vi "map modbus addresses test.vi"() -> ()   [LabVIEW 2013, in "Modbus Slave tests.lvlib"]
uses:
  Modbus Slave tests.lvlib
  configuration/Modbus Slave configuration.lvclass
  configuration/modbus mapping behavior.ctl
  <vilib>/NI/Tag Bus Module Framework/channel/channel classification.ctl
  <vilib>/NI/Tag Bus/tag/Data Type.ctl
  module channel/data bank type.ctl
  module channel/Modbus Module Channel.lvclass
  <vilib>/NI/Tag Bus/tag/tag descriptor.lvclass/tag descriptor.ctl
  <vilib>/NI/Tag Bus Module Framework/channel/TBM channel.lvclass/TBM channel.ctl
  module channel/Modbus Module Channel.lvclass/Modbus Module Channel.ctl
  configuration/Modbus Slave configuration.lvclass/Modbus Slave configuration.ctl
  <vilib>/NI/Tag Bus/tag/write tag name.vi
  <vilib>/NI/Tag Bus Module Framework/channel/Write channel classification.vi
  <vilib>/NI/Tag Bus/tag/write data type.vi
  module channel/Write modbus type.vi
  module channel/Write starting address.vi
  module channel/Write subindex (bool).vi
  <vilib>/NI/Tag Bus/tag/read tag name.vi
  <vilib>/NI/Tag Bus Module Framework/channel/Read channel classification.vi
  <vilib>/NI/Tag Bus/tag/read data type.vi
  module channel/Read modbus type.vi
  module channel/Read starting address.vi
  module channel/Read subindex (bool).vi
  <vilib>/NI/Tag Bus Module Framework/channel/TBM channel.lvclass
  <vilib>/NI/Tag Bus/tag/tag descriptor.lvclass
panel:
  in  "CSV Test File Path":path
  out "error out":errorcluster
  out "OK":bool
  in  "error in":errorcluster
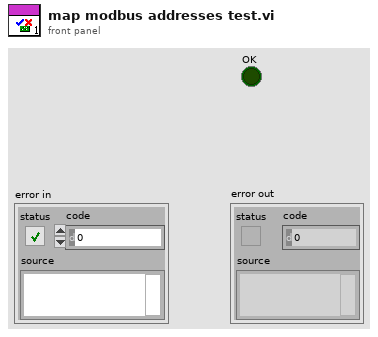
[diagram p1: front panel]
types:
  T1 = typedef "TBM channel.lvclass/channel classification.ctl" = enum16{"input data", "output data", "processing parameter", "processing result"}
  T2 = typedef "tag bus.lvlib/tag descriptor.lvclass/Data Type.ctl" = enum16{"Double", "Single", "I64", "I32", "I16", "I8", "U64", "U32", "U16", "U8", "Boolean", "String", "Array of Double", "Array of Single", "Array of I64", "Array of I32", "Array of I16", "Array of I8", "Array of U64", "Array of U32", "Array of U16", "Array of U8", "Array of Boolean", "Array of String"}
  T3 = typedef "Modbus Module Channel.lvclass/data bank type.ctl" = enum16{"coils", "discrete inputs", "input registers", "holding registers"}
  T4 = cluster{"name":string, "channel classification":T1, "data type":T2, "modbus type":T3, "starting address":u16, "subindex (bool)":i32}[]
  T5 = typedef "Modbus Slave configuration.lvclass/modbus mapping behavior.ctl" = enum16{"custom", "optimized"}
  T6 = cluster{"name":string, "channel classification":T1, "data type":T2, "modbus type":T3, "starting address":u16, "subindex (bool)":i32}
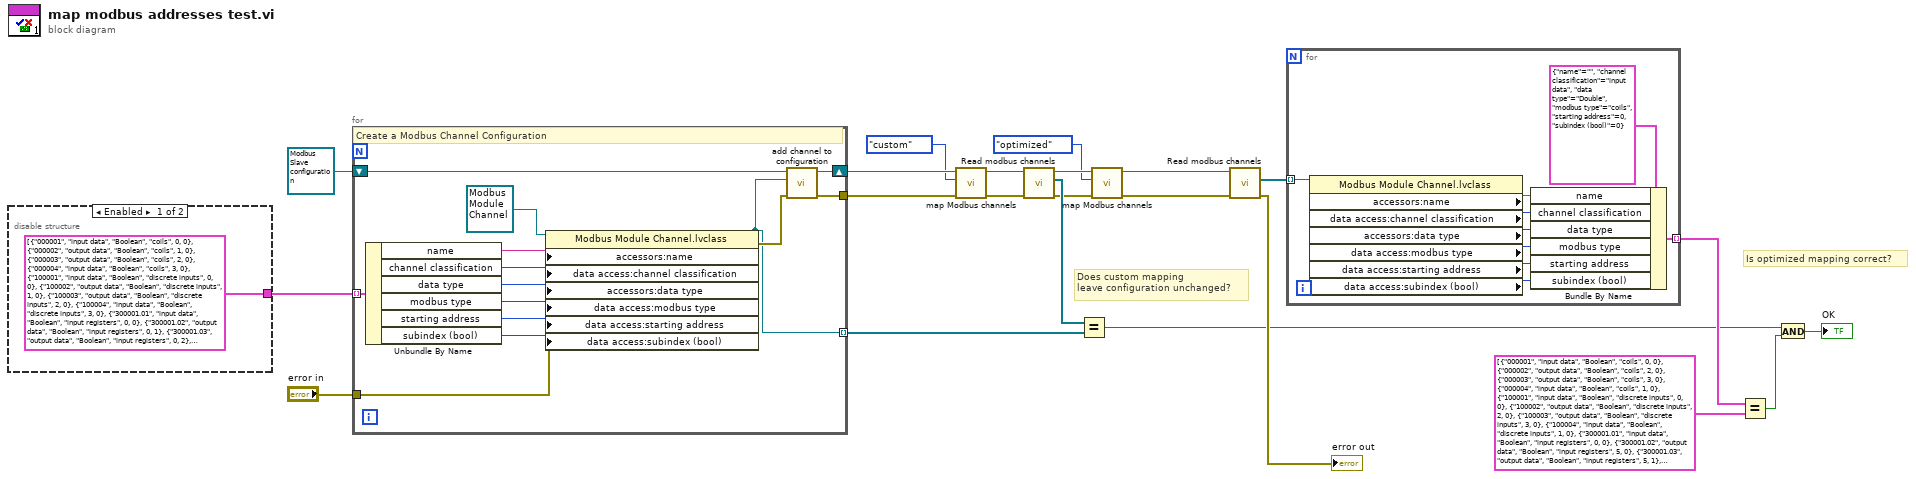
[diagram p0: block diagram]
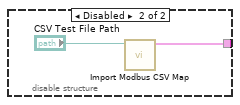
[diagram p2: hidden frame]
diagram:
  # "Is optimized mapping correct?"
  # "Does custom mapping\nleave configuration unchanged?"
  n1 = disable-structure shown="Enabled" {
    disable-tunnel: [T4 [{"name"="000001", "channel classification"=enum."input data", "data type"=enum."Boolean", "modbus type"=enum."coils", "starting address"=0, "subindex (bool)"=0}, {"name"="000002", "channel classification"=enum."output data", "data type"=enum."Boolean", "modbus type"=enum."coils", "starting address"=1, "subindex (bool)"=0}, {"name"="000003", "channel classification"=enum."output data", "data type"=enum."Boolean", "modbus type"=enum."coils", "starting address"=2, "subindex (bool)"=0}, {"name"="000004", "channel classification"=enum."input data", "data type"=enum."Boolean", "modbus type"=enum."coils", "starting address"=3, "subindex (bool)"=0}, {"name"="100001", "channel classification"=enum."input data", "data type"=enum."Boolean", "modbus type"=enum."discrete inputs", "starting address"=0, "subindex (bool)"=0}, {"name"="100002", "channel classification"=enum."output data", "data type"=enum."Boolean", "modbus type"=enum."discrete inputs", "starting address"=1, "subindex (bool)"=0}, {"name"="100003", "channel classification"=enum."output data", "data type"=enum."Boolean", "modbus type"=enum."discrete inputs", "starting address"=2, "subindex (bool)"=0}, {"name"="100004", "channel classification"=enum."input data", "data type"=enum."Boolean", "modbus type"=enum."discrete inputs", "starting address"=3, "subindex (bool)"=0}, {"name"="300001.01", "channel classification"=enum."input data", "data type"=enum."Boolean", "modbus type"=enum."input registers", "starting address"=0, "subindex (bool)"=0}, {"name"="300001.02", "channel classification"=enum."output data", "data type"=enum."Boolean", "modbus type"=enum."input registers", "starting address"=0, "subindex (bool)"=1}, {"name"="300001.03", "channel classification"=enum."output data", "data type"=enum."Boolean", "modbus type"=enum."input registers", "starting address"=0, "subindex (bool)"=2}, {"name"="300001.04", "channel classification"=enum."input data", "data type"=enum."Boolean", "modbus type"=enum."input registers", "starting address"=0, "subindex (bool)"=3}, {"name"="300001", "channel classification"=enum."input data", "data type"=enum."Single", "modbus type"=enum."input registers", "starting address"=0, "subindex (bool)"=0}, {"name"="300002", "channel classification"=enum."output data", "data type"=enum."Single", "modbus type"=enum."input registers", "starting address"=1, "subindex (bool)"=0}, {"name"="300003", "channel classification"=enum."output data", "data type"=enum."Single", "modbus type"=enum."input registers", "starting address"=2, "subindex (bool)"=0}, {"name"="300004", "channel classification"=enum."input data", "data type"=enum."Single", "modbus type"=enum."input registers", "starting address"=3, "subindex (bool)"=0}, {"name"="400001.01", "channel classification"=enum."input data", "data type"=enum."Boolean", "modbus type"=enum."holding registers", "starting address"=0, "subindex (bool)"=0}, {"name"="400001.02", "channel classification"=enum."output data", "data type"=enum."Boolean", "modbus type"=enum."holding registers", "starting address"=0, "subindex (bool)"=1}, {"name"="400001.03", "channel classification"=enum."output data", "data type"=enum."Boolean", "modbus type"=enum."holding registers", "starting address"=0, "subindex (bool)"=2}, {"name"="400001.04", "channel classification"=enum."input data", "data type"=enum."Boolean", "modbus type"=enum."holding registers", "starting address"=0, "subindex (bool)"=3}, {"name"="400001", "channel classification"=enum."input data", "data type"=enum."Double", "modbus type"=enum."holding registers", "starting address"=0, "subindex (bool)"=0}, {"name"="400002", "channel classification"=enum."output data", "data type"=enum."Double", "modbus type"=enum."holding registers", "starting address"=1, "subindex (bool)"=0}, {"name"="400003", "channel classification"=enum."output data", "data type"=enum."Double", "modbus type"=enum."holding registers", "starting address"=2, "subindex (bool)"=0}, {"name"="400004", "channel classification"=enum."input data", "data type"=enum."Double", "modbus type"=enum."holding registers", "starting address"=3, "subindex (bool)"=0}] ("Modbus address map 2") w25] -> w2
    frame Enabled {
    }
    frame Disabled {
      n2 = call "Import Modbus CSV Map.vi"("CSV Test File Path"="CSV Test File Path") -> ("Modbus address map"=w25:T4)  [unwired: 10 in]
    }
  }
  n3 = for {
    shift-right: [w29] -> w20
    shift-left: refnum<class "Modbus Slave configuration.lvclass"> refnum ("Modbus Slave configuration") -> [w31]
    tunnel: w2 -> [w38] mode=indexing
    tunnel: "error in" -> [w28]
    tunnel: [w27] -> w19
    tunnel: [w26] -> w14 mode=indexing
    # "Create a Modbus Channel Configuration"
    n4 = Unbundle By Name(w38) -> ("name"=w32:string, "channel classification"=w33:T1, "data type"=w34:T2, "modbus type"=w35:T3, "starting address"=w36:u16, "subindex (bool)"=w37:i32)
    n5 = property class="Modbus Module Channel.lvclass"(reference=refnum<class "Modbus Module Channel.lvclass"> refnum ("Modbus Module Channel.lvclass"), error in=w28, "accessors:name"=w32, "data access:channel classification"=w33, "accessors:data type"=w34, "data access:modbus type"=w35, "data access:starting address"=w36, "data access:subindex (bool)"=w37) -> (reference out=w26:refnum<class "Modbus Module Channel.lvclass">, error out=w30:errorcluster)
    n6 = call "add channel to configuration.vi"("error in"=w30, "Modbus Module Channel.lvclass"=w26, "Modbus Slave configuration in"=w31) -> ("error out"=w27:errorcluster, "Modbus Slave configuration out"=w29:refnum<class "Modbus Slave configuration.lvclass">)  [unwired: 7 in]
  }
  n7 = call "map Modbus channels.vi"("error in"=w19, "mapping"=modbus_mapping_behavior."custom", "Modbus Slave configuration in"=w20) -> ("error out"=w16:errorcluster, "Modbus Slave configuration out"=w17:refnum<class "Modbus Slave configuration.lvclass">)  [unwired: 7 in]
  n8 = call "Read modbus channels.vi"("error in"=w16, "Modbus Slave configuration in"=w17) -> ("error out"=w12:errorcluster, "modbus channels"=w15:refnum<class "Modbus Module Channel.lvclass">[], "Modbus Slave configuration out"=w13:refnum<class "Modbus Slave configuration.lvclass">)  [unwired: 7 in]
  n9 = Equal?(x=w15, y=w14) -> (x = y?=w5:bool)
  n10 = call "map Modbus channels.vi"("error in"=w12, "mapping"=modbus_mapping_behavior."optimized", "Modbus Slave configuration in"=w13) -> ("error out"=w9:errorcluster, "Modbus Slave configuration out"=w10:refnum<class "Modbus Slave configuration.lvclass">)  [unwired: 7 in]
  n11 = call "Read modbus channels.vi"("error in"=w9, "Modbus Slave configuration in"=w10) -> ("error out"=→"error out":errorcluster, "modbus channels"=w8:refnum<class "Modbus Module Channel.lvclass">[])  [unwired: 7 in, 1 out]
  n12 = for {
    tunnel: w8 -> [w48] mode=indexing
    tunnel: [w40] -> w6 mode=indexing
    n13 = property class="Modbus Module Channel.lvclass"(reference=w48) -> ("accessors:name"=w46:string, "data access:channel classification"=w45:T1, "accessors:data type"=w44:T2, "data access:modbus type"=w43:T3, "data access:starting address"=w42:u16, "data access:subindex (bool)"=w41:i32)  [unwired: 1 in, 2 out]
    n14 = Bundle By Name(cluster=T6 {"name"="", "channel classification"=enum."input data", "data type"=enum."Double", "modbus type"=enum."coils", "starting address"=0, "subindex (bool)"=0}, "name"=w46, "channel classification"=w45, "data type"=w44, "modbus type"=w43, "starting address"=w42, "subindex (bool)"=w41) -> (w40:T6)
  }
  n15 = Equal?(x=w6, y=T4 [{"name"="000001", "channel classification"=enum."input data", "data type"=enum."Boolean", "modbus type"=enum."coils", "starting address"=0, "subindex (bool)"=0}, {"name"="000002", "channel classification"=enum."output data", "data type"=enum."Boolean", "modbus type"=enum."coils", "starting address"=2, "subindex (bool)"=0}, {"name"="000003", "channel classification"=enum."output data", "data type"=enum."Boolean", "modbus type"=enum."coils", "starting address"=3, "subindex (bool)"=0}, {"name"="000004", "channel classification"=enum."input data", "data type"=enum."Boolean", "modbus type"=enum."coils", "starting address"=1, "subindex (bool)"=0}, {"name"="100001", "channel classification"=enum."input data", "data type"=enum."Boolean", "modbus type"=enum."discrete inputs", "starting address"=0, "subindex (bool)"=0}, {"name"="100002", "channel classification"=enum."output data", "data type"=enum."Boolean", "modbus type"=enum."discrete inputs", "starting address"=2, "subindex (bool)"=0}, {"name"="100003", "channel classification"=enum."output data", "data type"=enum."Boolean", "modbus type"=enum."discrete inputs", "starting address"=3, "subindex (bool)"=0}, {"name"="100004", "channel classification"=enum."input data", "data type"=enum."Boolean", "modbus type"=enum."discrete inputs", "starting address"=1, "subindex (bool)"=0}, {"name"="300001.01", "channel classification"=enum."input data", "data type"=enum."Boolean", "modbus type"=enum."input registers", "starting address"=0, "subindex (bool)"=0}, {"name"="300001.02", "channel classification"=enum."output data", "data type"=enum."Boolean", "modbus type"=enum."input registers", "starting address"=5, "subindex (bool)"=0}, {"name"="300001.03", "channel classification"=enum."output data", "data type"=enum."Boolean", "modbus type"=enum."input registers", "starting address"=5, "subindex (bool)"=1}, {"name"="300001.04", "channel classification"=enum."input data", "data type"=enum."Boolean", "modbus type"=enum."input registers", "starting address"=0, "subindex (bool)"=1}, {"name"="300001", "channel classification"=enum."input data", "data type"=enum."Single", "modbus type"=enum."input registers", "starting address"=1, "subindex (bool)"=0}, {"name"="300002", "channel classification"=enum."output data", "data type"=enum."Single", "modbus type"=enum."input registers", "starting address"=6, "subindex (bool)"=0}, {"name"="300003", "channel classification"=enum."output data", "data type"=enum."Single", "modbus type"=enum."input registers", "starting address"=8, "subindex (bool)"=0}, {"name"="300004", "channel classification"=enum."input data", "data type"=enum."Single", "modbus type"=enum."input registers", "starting address"=3, "subindex (bool)"=0}, {"name"="400001.01", "channel classification"=enum."input data", "data type"=enum."Boolean", "modbus type"=enum."holding registers", "starting address"=0, "subindex (bool)"=0}, {"name"="400001.02", "channel classification"=enum."output data", "data type"=enum."Boolean", "modbus type"=enum."holding registers", "starting address"=9, "subindex (bool)"=0}, {"name"="400001.03", "channel classification"=enum."output data", "data type"=enum."Boolean", "modbus type"=enum."holding registers", "starting address"=9, "subindex (bool)"=1}, {"name"="400001.04", "channel classification"=enum."input data", "data type"=enum."Boolean", "modbus type"=enum."holding registers", "starting address"=0, "subindex (bool)"=1}, {"name"="400001", "channel classification"=enum."input data", "data type"=enum."Double", "modbus type"=enum."holding registers", "starting address"=1, "subindex (bool)"=0}, {"name"="400002", "channel classification"=enum."output data", "data type"=enum."Double", "modbus type"=enum."holding registers", "starting address"=10, "subindex (bool)"=0}, {"name"="400003", "channel classification"=enum."output data", "data type"=enum."Double", "modbus type"=enum."holding registers", "starting address"=14, "subindex (bool)"=0}, {"name"="400004", "channel classification"=enum."input data", "data type"=enum."Double", "modbus type"=enum."holding registers", "starting address"=5, "subindex (bool)"=0}] ("Modbus address map 2")) -> (x = y?=w4:bool)
  n16 = And(x=w5, y=w4) -> (x .and. y?=→"OK":bool)
